vi "Read Test Executive Ref.vi"(11 "Test Executive Builder Model in":refnum<class "Test Executive Builder Model.lvclass">) -> (2 "Test Executive Ref":refnum<data-value>, 3 "Test Executive Builder Model out":refnum<class "Test Executive Builder Model.lvclass">)   [LabVIEW 2017, in "Test Executive Builder Model.lvclass"]
uses:
  Test Executive Builder Model.lvclass
  <vilib>/gpm_packages/@cs/test-executive/Source/Test Executive/ITestExecutive/ITest Executive.lvclass
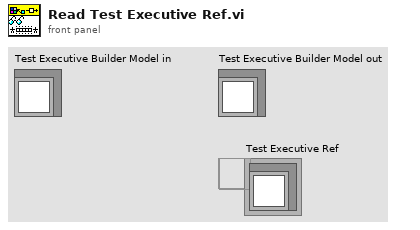
[diagram p1: front panel]
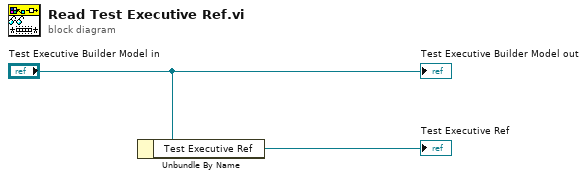
[diagram p0: block diagram]
diagram:
  n1 = Unbundle By Name("Test Executive Builder Model in") -> ("Test Executive Ref"=→"Test Executive Ref":refnum<data-value>)
  "Test Executive Builder Model out" <- "Test Executive Builder Model in"
